vi "Run Testing Test Iteration.vi"(7 "Number of Concurrent Calls (4)":i32=4, 8 "error in (no error)":errorcluster, 11 "gRPC ID":T2) -> (0 "error out":errorcluster, 3 "Timing Statistics":T1)   [LabVIEW 2021]
uses:
  <vilib>/gRPC/LabVIEW gRPC Library/Shared/grpcId.ctl
  TYPEDEF - Timing Statistics.ctl
  gRPC/test_service_client/RPC Messages/test_service_Method1Request.ctl
  gRPC/test_service_client/RPC Messages/test_service_Method2Request.ctl
  gRPC/test_service_client/RPC Messages/test_service_Method3Request.ctl
  gRPC/test_service_client/RPC Messages/test_service_Method4Request.ctl
  gRPC/test_service_client/test_service_client.lvlib
  <vilib>/gRPC/LabVIEW gRPC Library/grpc-lvsupport-release.lvlib
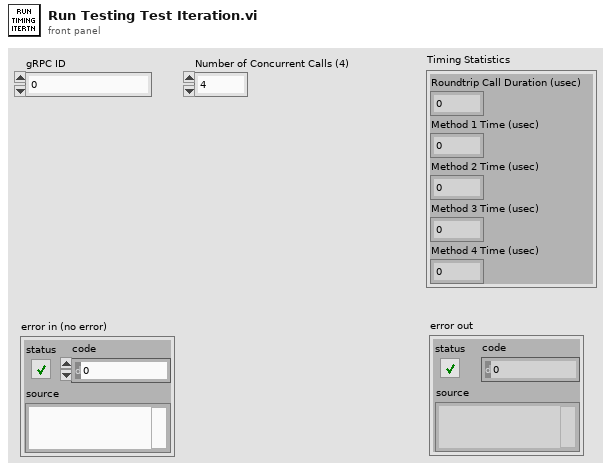
[diagram p1: front panel]
types:
  T1 = typedef "TYPEDEF - Timing Statistics.ctl" = cluster{"Roundtrip Call Duration (usec)":u64, "Method 1 Time (usec)":u64, "Method 2 Time (usec)":u64, "Method 3 Time (usec)":u64, "Method 4 Time (usec)":u64}
  T2 = typedef "grpc-lvsupport-release.lvlib/grpcId.ctl" = u64
  T3 = typedef "test_service_client.lvlib/test_service_Method4Request.ctl" = cluster{"timestamp":u64}
  T4 = typedef "test_service_client.lvlib/test_service_Method3Request.ctl" = cluster{"timestamp":u64}
  T5 = typedef "test_service_client.lvlib/test_service_Method2Request.ctl" = cluster{"timestamp":u64}
  T6 = typedef "test_service_client.lvlib/test_service_Method1Request.ctl" = cluster{"timestamp":u64}
  T7 = typedef "test_service_client.lvlib/test_service_Method1Response.ctl" = cluster{"timestamp_request":u64, "timestamp":u64}
  T8 = typedef "test_service_client.lvlib/test_service_Method2Response.ctl" = cluster{"timestamp_request":u64, "timestamp":u64}
  T9 = typedef "test_service_client.lvlib/test_service_Method3Response.ctl" = cluster{"timestamp_request":u64, "timestamp":u64}
  T10 = typedef "test_service_client.lvlib/test_service_Method4Response.ctl" = cluster{"timestamp_request":u64, "timestamp":u64}
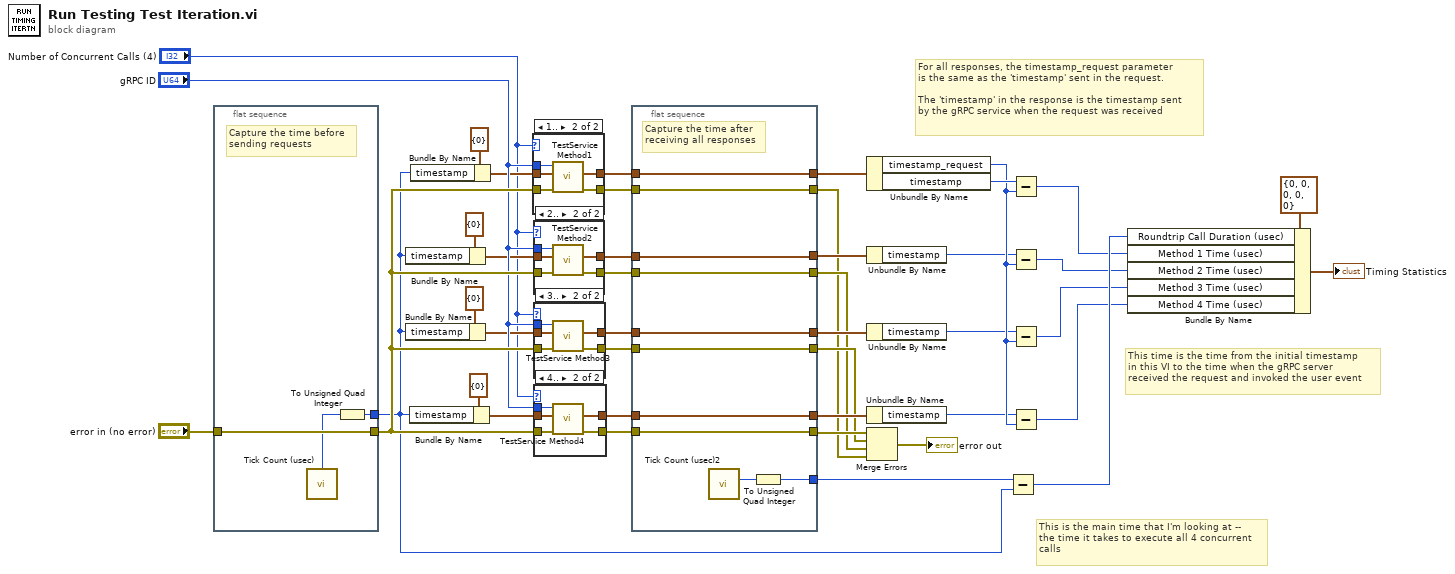
[diagram p0: block diagram]
diagram:
  # "This time is the time from the initial timestamp\nin this VI to the time when the gRPC server\nreceived the request and invoked the user event"
  # "This is the main time that I'm looking at --\nthe time it takes to execute all 4 concurrent\ncalls"
  # "For all responses, the timestamp_request parameter\nis the same as the 'timestamp' sent in the request.\n\nThe 'timestamp' in the response is the timestamp sent\nby the gRPC service when the request was received"
  n1 = flat-sequence {
    tunnel: [w44] -> w5
    tunnel: [w46] -> w33
    tunnel: "error in (no error)" -> [w46]
    frame #0 {
      # "Capture the time before\nsending requests"
      n2 = call "Tick Count (usec)"() -> ("Tick Count(uSec)"=w45:u32)
      n3 = To Unsigned Quad Integer(1:w45) -> (0:w44:u64)
    }
  }
  n4 = Bundle By Name(cluster=T5 {"timestamp"=0} ("Request Data"), "timestamp"=w5) -> (w4:T5)
  n5 = Bundle By Name(cluster=T4 {"timestamp"=0} ("Request Data"), "timestamp"=w5) -> (w3:T4)
  n6 = Bundle By Name(cluster=T3 {"timestamp"=0} ("Request Data"), "timestamp"=w5) -> (w2:T3)
  n7 = Bundle By Name(cluster=T6 {"timestamp"=0} ("Request Data"), "timestamp"=w5) -> (w9:T6)
  n8 = case shown="1.." "Number of Concurrent Calls (4)" {
    tunnel: [w47 w52] -> w42
    tunnel: [_ w51] -> w38
    tunnel: w33 -> [w47 w50]
    tunnel: "gRPC ID" -> [_ w49]
    tunnel: w9 -> [_ w48]
    frame 0, Default {
    }
    frame 1.. {
      n9 = call "TestService Method1.vi"("error in"=w50, "Request Data"=w48, "gRPC ID"=w49) -> ("error out"=w52:errorcluster, "Response Data"=w51:T7)  [unwired: 6 in, 1 out]
    }
  }
  n10 = case shown="2.." "Number of Concurrent Calls (4)" {
    tunnel: [w53 w58] -> w41
    tunnel: [_ w57] -> w37
    tunnel: w33 -> [w53 w56]
    tunnel: "gRPC ID" -> [_ w55]
    tunnel: w4 -> [_ w54]
    frame 0, Default {
    }
    frame 2.. {
      n11 = call "TestService Method2.vi"("error in"=w56, "Request Data"=w54, "gRPC ID"=w55) -> ("error out"=w58:errorcluster, "Response Data"=w57:T8)  [unwired: 6 in, 1 out]
    }
  }
  n12 = case shown="3.." "Number of Concurrent Calls (4)" {
    tunnel: [w59 w64] -> w39
    tunnel: [_ w63] -> w36
    tunnel: w33 -> [w59 w62]
    tunnel: "gRPC ID" -> [_ w61]
    tunnel: w3 -> [_ w60]
    frame 0, Default {
    }
    frame 3.. {
      n13 = call "TestService Method3.vi"("error in"=w62, "Request Data"=w60, "gRPC ID"=w61) -> ("error out"=w64:errorcluster, "Response Data"=w63:T9)  [unwired: 6 in, 1 out]
    }
  }
  n14 = case shown="4.." "Number of Concurrent Calls (4)" {
    tunnel: [w65 w70] -> w40
    tunnel: [_ w69] -> w35
    tunnel: w33 -> [w65 w68]
    tunnel: "gRPC ID" -> [_ w67]
    tunnel: w2 -> [_ w66]
    frame 0, Default {
    }
    frame 4.. {
      n15 = call "TestService Method4.vi"("error in"=w68, "Request Data"=w66, "gRPC ID"=w67) -> ("error out"=w70:errorcluster, "Response Data"=w69:T10)  [unwired: 6 in, 1 out]
    }
  }
  n16 = flat-sequence {
    tunnel: [w71] -> w16
    tunnel: [w79] -> w27
    tunnel: w40 -> [w79]
    tunnel: [w78] -> w26
    tunnel: w39 -> [w78]
    tunnel: [w77] -> w25
    tunnel: w41 -> [w77]
    tunnel: [w76] -> w24
    tunnel: w42 -> [w76]
    tunnel: w38 -> [w75]
    tunnel: w37 -> [w74]
    tunnel: w36 -> [w73]
    tunnel: w35 -> [w72]
    tunnel: [w75] -> w31
    tunnel: [w74] -> w30
    tunnel: [w73] -> w28
    tunnel: [w72] -> w29
    frame #0 {
      # "Capture the time after \nreceiving all responses"
      n17 = call "Tick Count (usec)2"() -> ("Tick Count(uSec)"=w80:u32)
      n18 = To Unsigned Quad Integer(1:w80) -> (0:w71:u64)
    }
  }
  n19 = Unbundle By Name(w31) -> ("timestamp_request"=w21:u64, "timestamp"=w22:u64)
  n20 = Unbundle By Name(w30) -> ("timestamp"=w18:u64)
  n21 = Unbundle By Name(w28) -> ("timestamp"=w19:u64)
  n22 = Unbundle By Name(w29) -> ("timestamp"=w20:u64)
  n23 = Merge Errors(w27, w26, w25, w24) -> (→"error out":errorcluster)
  n24 = Subtract(x=w16, y=w5) -> (x-y=w15:u64)
  n25 = Subtract(x=w22, y=w21) -> (x-y=w14:u64)
  n26 = Subtract(x=w18, y=w21) -> (x-y=w13:u64)
  n27 = Subtract(x=w19, y=w21) -> (x-y=w12:u64)
  n28 = Subtract(x=w20, y=w21) -> (x-y=w11:u64)
  n29 = Bundle By Name(cluster=T1 {"Roundtrip Call Duration (usec)"=0, "Method 1 Time (usec)"=0, "Method 2 Time (usec)"=0, "Method 3 Time (usec)"=0, "Method 4 Time (usec)"=0} ("Timing Statistics"), "Roundtrip Call Duration (usec)"=w15, "Method 1 Time (usec)"=w14, "Method 2 Time (usec)"=w13, "Method 3 Time (usec)"=w12, "Method 4 Time (usec)"=w11) -> (→"Timing Statistics":T1)
